vi "run.vi"() -> ()   [LabVIEW 2010]
uses:
  references.ctl
panel:
  out "errors":string
  out "error out":errorcluster
  out "Total":i32
  out "Results":string
  out "Progress":i32(slide) scale=0.0..3108.0
  out "Completed":i32 max=405
  in  "error in (no error)":errorcluster
  in  "Path":path=path "C:/test"
  # "of"
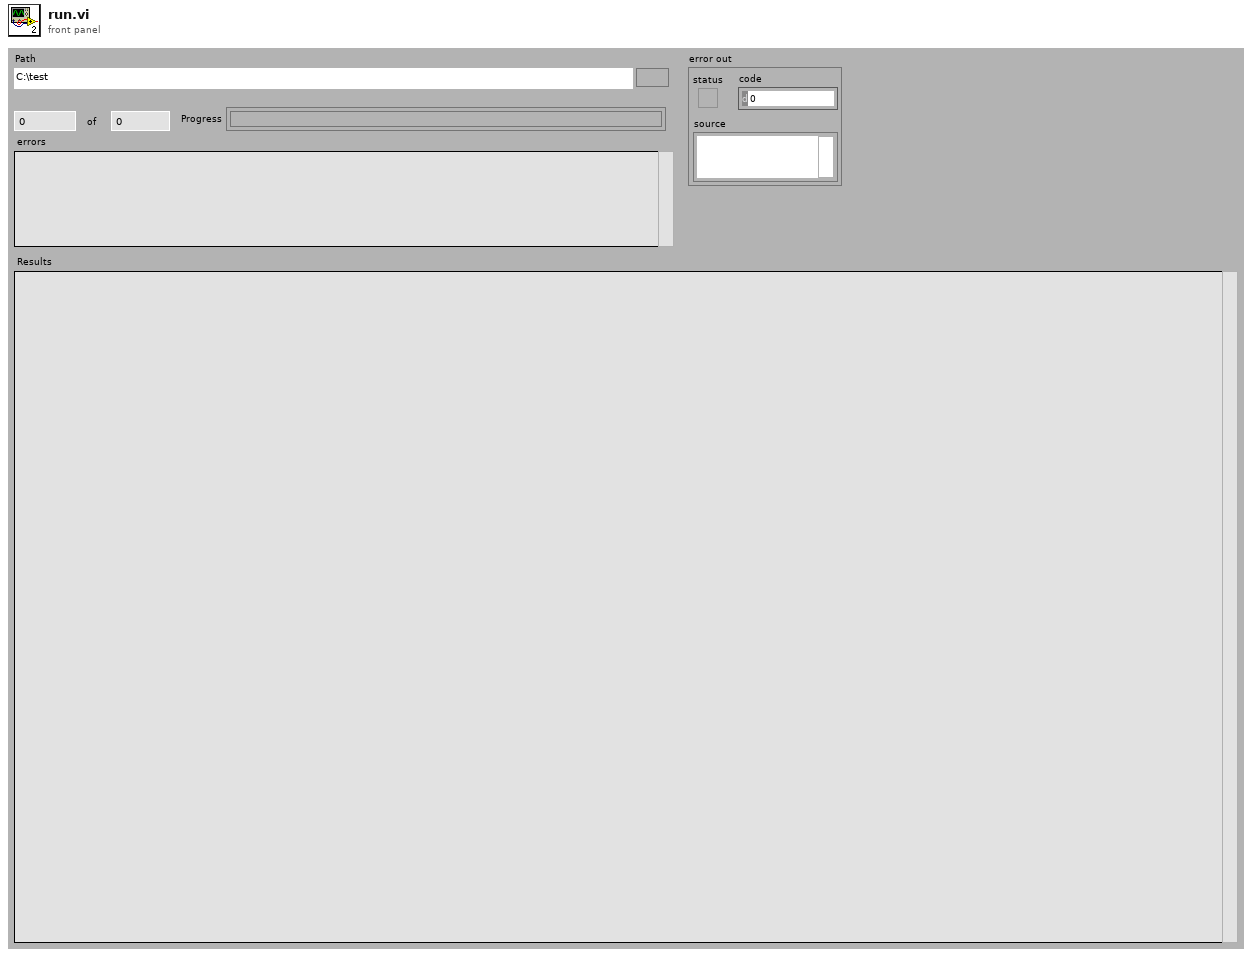
[diagram p1: front panel]
types:
  T1 = typedef "references.ctl" = cluster{"errors":refnum<vi>, "Results":refnum<vi>, "Completed":refnum<vi>}
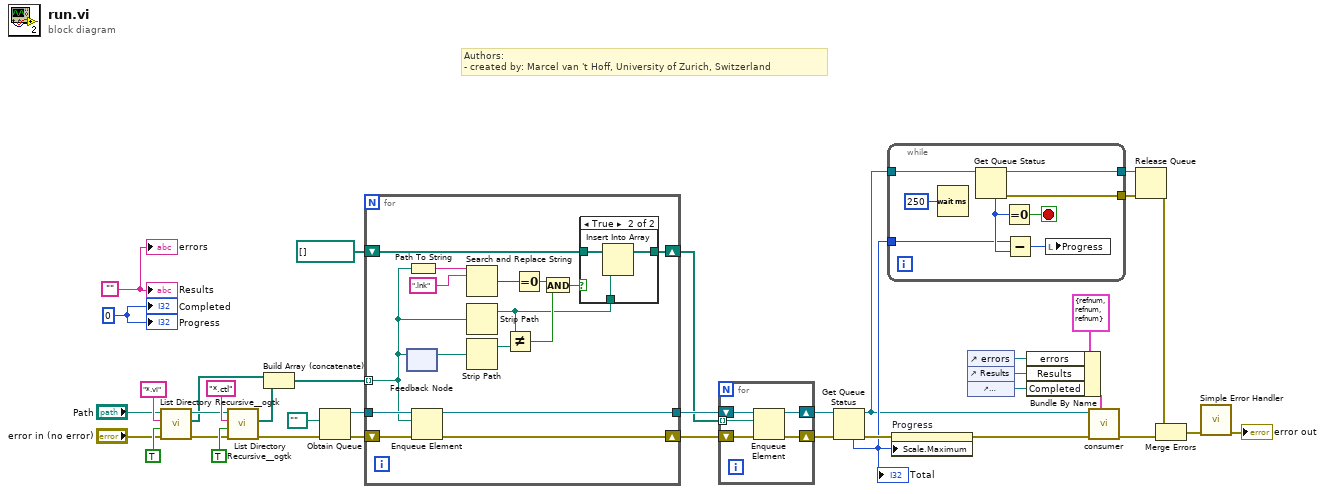
[diagram p0: block diagram]
diagram:
  w31 = 0 ("Completed")
  w29 = ""
  # "Authors: \n- created by: Marcel van 't Hoff, University of Zurich, Switzerland"
  n1 = call <userlib>:"List Directory Recursive__ogtk.vi"("error in (no error)"="error in (no error)", "Treat llb files as directories? (FALSE)"=TRUE, "pattern"="*.vi", "Path"="Path") -> ("error out"=w33:errorcluster, "file paths"=w28:path[], "dup Path"=w34:path)  [unwired: 4 in, 1 out]
  n2 = call <userlib>:"List Directory Recursive__ogtk.vi"("error in (no error)"=w33, "Treat llb files as directories? (FALSE)"=TRUE, "pattern"="*.ctl", "Path"=w34) -> ("error out"=w30:errorcluster, "file paths"=w27:path[])  [unwired: 4 in, 2 out]
  n3 = Build Array (concatenate)(w28, w27) -> (w15:path[])
  n4 = Obtain Queue(element data type=path "" ("Path"), error in (no error)=w30) -> (queue out=w25:refnum<queue>, error out=w24:errorcluster)  [unwired: 3 in, 1 out]
  n5 = for {
    tunnel: w15 -> [w50] mode=indexing
    tunnel: w25 -> [w54]
    shift-right: [w43] -> w12
    shift-left: w24 -> [w53]
    tunnel: [w44] -> w11
    shift-right: [w40] -> w10
    shift-left: path[] [] -> [w41]
    n6 = feedback-in #1(w50) -> ()
    n7 = feedback #1() -> (w52:path)  [unwired: 1 in]
    n8 = Path To String(path=w50) -> (string=w49:string)
    n9 = Enqueue Element(queue=w54, element=w50, error in (no error)=w53) -> (queue out=w44:refnum<queue>, error out=w43:errorcluster)  [unwired: 1 in, 1 out]
    n10 = Search and Replace String(input string=w49, search string=".lnk") -> (number of replacements=w46:i32)  [unwired: 6 in, 3 out]
    n11 = Strip Path(path=w50) -> (stripped path=w39:path)  [unwired: 1 out]
    n12 = Strip Path(path=w52) -> (stripped path=w51:path)  [unwired: 1 out]
    n13 = Not Equal?(x=w39, y=w51) -> (x != y?=w47:bool)
    n14 = Equal To 0?(x=w46) -> (x = 0?=w45:bool)
    n15 = And(x=w45, y=w47) -> (x .and. y?=w42:bool)
    n16 = case shown="True" w42 {
      tunnel: w41 -> [w55 w58]
      tunnel: [w55 w57] -> w40
      tunnel: w39 -> [_ w56]
      frame False {
      }
      frame True {
        n17 = Insert Into Array(array=w58, new element=w56) -> (w57:path[])  [unwired: 1 in]
      }
    }
  }
  n18 = for {
    shift-right: [w60] -> w8
    shift-left: w12 -> [w61]
    tunnel: w10 -> [w59] mode=indexing
    shift-right: [w62] -> w9
    shift-left: w11 -> [w63]
    n19 = Enqueue Element(queue=w63, element=w59, error in (no error)=w61) -> (queue out=w62:refnum<queue>, error out=w60:errorcluster)  [unwired: 1 in, 1 out]
  }
  n20 = Get Queue Status(queue=w9, error in (no error)=w8) -> (queue out=w4:refnum<queue>, error out=w7:errorcluster, # elements in queue=w5:i32)  [unwired: 1 in, 5 out]
  "Total" <- w5
  n21 = while {
    tunnel: w4 -> [w71]
    tunnel: [w69] -> w23
    tunnel: [w68] -> w22
    tunnel: w5 -> [w64]
    stop <- w70 stop-if-true
    n22 = Wait (ms)(milliseconds to wait=u32 250) -> ()  [unwired: 1 out]
    n23 = Get Queue Status(queue=w71) -> (queue out=w69:refnum<queue>, error out=w68:errorcluster, # elements in queue=w66:i32)  [unwired: 2 in, 5 out]
    n24 = Equal To 0?(x=w66) -> (x = 0?=w70:bool)
    n25 = Subtract(x=w64, y=w66) -> (x-y=w65:i32)
    n26 = local write "Progress"(w65) -> ()
  }
  n27 = property on="Progress" class="Slide (strict)"(error in=w7, "Scale.Maximum"=w5) -> (error out=w6:errorcluster)  [unwired: 1 in, 1 out]
  n28 = control-ref of="errors"() -> (w20:refnum<vi>)
  n29 = control-ref of="Results"() -> (w19:refnum<vi>)
  n30 = control-ref of="Completed"() -> (w18:refnum<vi>)
  n31 = Bundle By Name(cluster=T1 {"errors"=refnum, "Results"=refnum, "Completed"=refnum} ("Cluster"), "errors"=w20, "Results"=w19, "Completed"=w18) -> (w3:T1)
  n32 = call "consumer.vi"("Cluster"=w3, "error in"=w6, "queue in"=w4) -> ("error out"=w16:errorcluster)  [unwired: 7 in, 1 out]
  n33 = Release Queue(queue=w23, error in (no error)=w22) -> (error out=w17:errorcluster)  [unwired: 1 in, 2 out]
  n34 = Merge Errors(w17, w16) -> (w2:errorcluster)
  n35 = call <vilib>:"Simple Error Handler.vi"("error in (no error)"=w2) -> ("error out"=→"error out":errorcluster)  [unwired: 4 in, 4 out]
  "Results" <- w29
  "Progress" <- w31
  "Completed" <- w31
  "errors" <- w29
